vi "GFITS_Parse_comment_single.vi"(9 "found":bool, 10 "comment in":string, 11 "value in":string) -> (0 "write?":bool, 2 "comment out":string, 3 "value out":string)   [LabVIEW 2016]
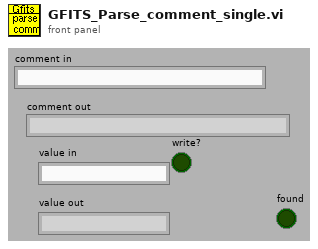
[diagram p1: front panel]
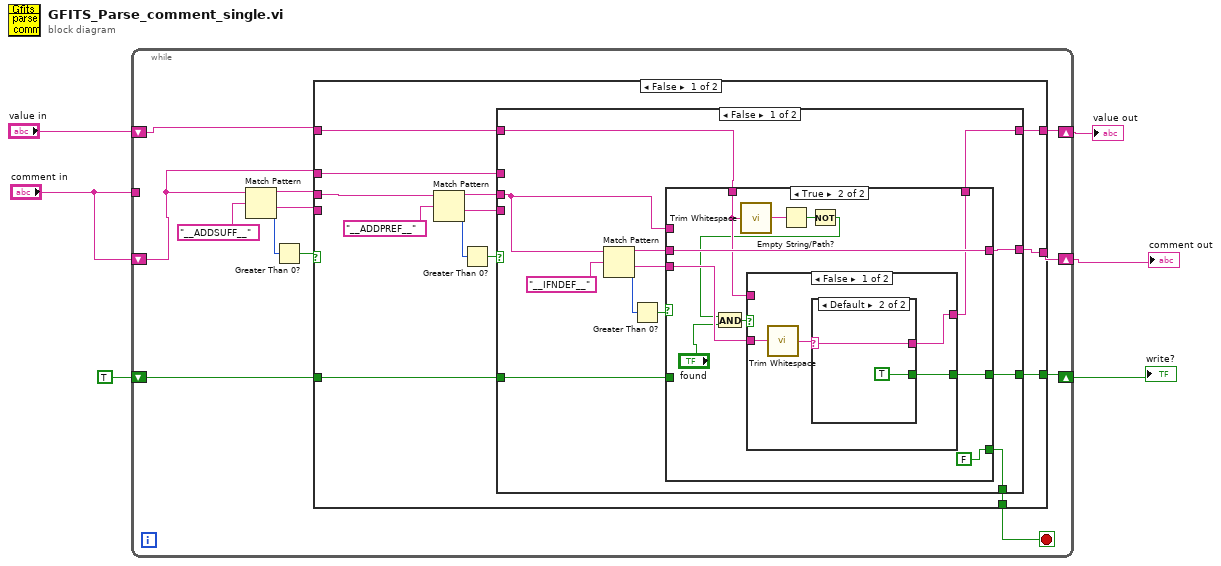
[diagram p0: block diagram]
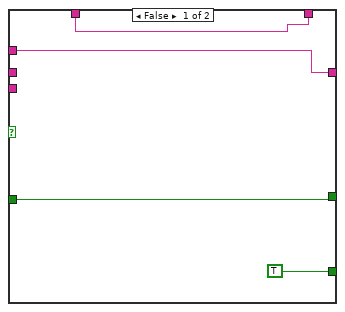
[diagram p2: hidden frame]
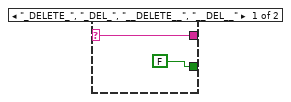
[diagram p3: hidden frame]
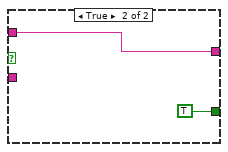
[diagram p4: hidden frame]
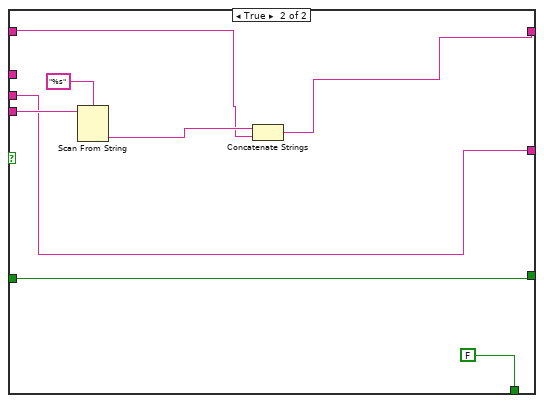
[diagram p5: hidden frame]
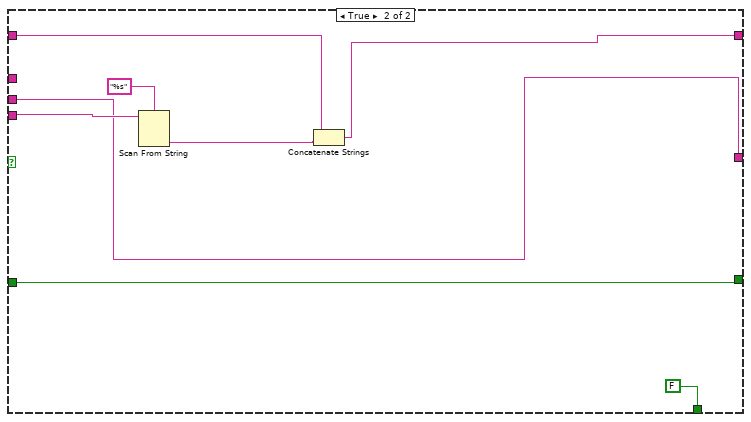
[diagram p6: hidden frame]
diagram:
  n1 = while {
    tunnel: "comment in" -> [_]
    shift-right: [w11] -> w4
    shift-left: "comment in" -> [w12]
    shift-right: [w9] -> w3
    shift-left: "value in" -> [w13]
    shift-right: [w8] -> w1
    shift-left: TRUE ("write?") -> [w7]
    stop <- w10 stop-if-true
    n2 = Match Pattern(string=w12, regular expression="__ADDSUFF__") -> (before substring=w14:string, after substring=w15:string, offset past match=w17:i32)  [unwired: 2 out]
    n3 = Greater Than 0?(x=w17) -> (x > 0?=w16:bool)
    n4 = case shown="False" w16 {
      tunnel: w15 -> [_ w84]
      tunnel: w12 -> [w26 _]
      tunnel: [w25 w81] -> w11
      tunnel: w13 -> [w28 w80]
      tunnel: [w24 w79] -> w9
      tunnel: w14 -> [w29 w81]
      tunnel: [w21 FALSE] -> w10
      tunnel: [w20 w77] -> w8
      tunnel: w7 -> [w19 w77]
      frame False {
        n5 = Match Pattern(string=w29, regular expression="__ADDPREF__") -> (before substring=w22:string, after substring=w23:string, offset past match=w30:i32)  [unwired: 2 out]
        n6 = Greater Than 0?(x=w30) -> (x > 0?=w27:bool)
        n7 = case shown="False" w27 {
          tunnel: w28 -> [w36 w72]
          tunnel: w26 -> [_ _]
          tunnel: [w38 w73] -> w25
          tunnel: [w35 w71] -> w24
          tunnel: w23 -> [_ w74]
          tunnel: w22 -> [w37 w73]
          tunnel: [w40 FALSE] -> w21
          tunnel: [w33 w69] -> w20
          tunnel: w19 -> [w32 w69]
          frame False {
            n8 = Match Pattern(string=w37, regular expression="__IFNDEF__") -> (before substring=w39:string, after substring=w34:string, offset past match=w42:i32)  [unwired: 2 out]
            n9 = Greater Than 0?(x=w42) -> (x > 0?=w41:bool)
            n10 = case shown="True" w41 {
              tunnel: [TRUE FALSE] -> w40
              tunnel: [w46 w57] -> w38
              tunnel: w39 -> [_ w57]
              tunnel: w37 -> [w46 _]
              tunnel: w36 -> [w45 w53]
              tunnel: [w45 w56] -> w35
              tunnel: w34 -> [_ w55]
              tunnel: [w44 w54] -> w33
              tunnel: w32 -> [w44 _]
              frame False {
              }
              frame True {
                n11 = call <vilib>:"Trim Whitespace.vi"("string"=w53) -> ("trimmed string"=w52:string)  [unwired: 1 in]
                n12 = Empty String/Path?(string/path=w52) -> (empty?=w50:bool)
                n13 = Not(x=w50) -> (.not. x?=w48:bool)
                n14 = And(x=w48, y="found") -> (x .and. y?=w49:bool)
                n15 = case shown="False" w49 {
                  tunnel: w53 -> [_ w68]
                  tunnel: [w60 w68] -> w56
                  tunnel: w55 -> [w62 _]
                  tunnel: [w59 TRUE ("write?")] -> w54
                  frame False {
                    n16 = call <vilib>:"Trim Whitespace.vi"("string"=w62) -> ("trimmed string"=w61:string)  [unwired: 1 in]
                    n17 = case shown="Default" w61 {
                      selector: w61 -> [w64 w66]
                      tunnel: [w64 w66] -> w60
                      tunnel: [FALSE ("write?") TRUE ("write?")] -> w59
                      frame "_DELETE_", "_DEL_", "__DELETE__", "__DEL__" {
                      }
                      frame Default {
                      }
                    }
                  }
                  frame True {
                  }
                }
              }
            }
          }
          frame True {
            n18 = Scan From String(format string="%s", input string=w74) -> (output 1=w75:string)  [unwired: 2 in, 4 out]
            n19 = Concatenate Strings(w75, w72) -> (w71:string)
          }
        }
      }
      frame True {
        n20 = Scan From String(format string="%s", input string=w84) -> (output 1=w82:string)  [unwired: 2 in, 4 out]
        n21 = Concatenate Strings(w80, w82) -> (w79:string)
      }
    }
  }
  "comment out" <- w4
  "value out" <- w3
  "write?" <- w1
